vi "Double FFT Mesurament RT with Frequency Linearization & BackNoise Remove Test.vi"() -> ()   [LabVIEW 2014]
uses:
  <vilib>/Platform/TimedLoop/XDataNode/timing_clust.ctl
  <vilib>/Platform/TimedLoop/XDataNode/nitl_modes.ctl
  <vilib>/Platform/TimedLoop/XDataNode/wakeup.ctl
  <vilib>/FPGAPlugInAG/sbRIO-9636/niLvFpga_Open_sbRIO-9636.vi
  <vilib>/rvi/interface/common/dynamic/niFpgaDynamicAddResources.vi
  <vilib>/FPGAPlugInAG/Dynamic/niLvFpga_Reset_Dynamic.vi
  <vilib>/Utility/error.llb/Error Cluster From Error Code.vi
  <vilib>/rvi/errors/niLvFpgaAdjustHostInterfaceError.vi
  <vilib>/rvi/interface/common/niFpgaWaitOnOcc.vi
  <vilib>/FPGAPlugInAG/Dynamic/niLvFpga_Run_Dynamic.vi
  <vilib>/FPGAPlugInAG/Dynamic/niLvFpga_Abort_Dynamic.vi
  <vilib>/FPGAPlugInAG/Dynamic/niLvFpga_Close_Dynamic.vi
  <vilib>/rvi/interface/nirviOpenFPGA/nirviOpenFPGA.xnode
  FPGA Bitfiles/LaserDistanceSen_FPGATarget_DoubleFFTMesuram_6dDziXQAIGE.lvbitx
  FPGA Target/Test VIs/Double FFT Mesurament Test with Background Noise Remove.vi
  <vilib>/rvi/interface/nirviMethod/nirviMethod.xnode
  <vilib>/rvi/interface/nirviReadWriteControl/nirviReadWriteControl.xnode
  <vilib>/Platform/TimedLoop/XDataNode/XDataNode.xnode
  <vilib>/rvi/interface/nirviCloseFPGA/nirviCloseFPGA.xnode
  <vilib>/FPGAPlugInAG/Dynamic/niLvFpga_ConfigureFifo_Dynamic.vi
  <vilib>/rvi/errors/niLvFpgaMergeErrorWithErrorCode.vi
  <vilib>/FPGAPlugInAG/Dynamic/niLvFpga_StartFifo_Dynamic.vi
  <vilib>/rvi/interface/Simulation/niFpgaSimulationCallBeginRW.vi
  <vilib>/FPGAPlugInAG/Dynamic/niLvFpga_ReadFifo_Dynamic.vi
  <vilib>/Platform/TimedLoop/XDataNode/XDNodeRunTimeDep.lvlib
  NiFpgaLv.dll
panel:
  in  "polynomial order":i32=3
  in  "side points":i32=6
  out "2^(n-bit) misure mediate":dbl
  in  "n-bit":i32=10
  in  "SubtractionType":T1(ring)=enum."StartingCurve"
  out "Fondo Signal":dbl[](graph)
  in  "LowPass Filter: Low cutoff frequency":dbl=20000.0 format="%#_13g"
  in  "PolyFitting: Poly Grade":dbl=12.0
  in  "Scale Factor Rising":dbl=0.5
  out "2) Std Dev":dbl
  out "1) Std Dev":dbl
  in  "Scale Factor Falling":dbl=0.5
  in  "Triangolo dritto":bool
  in  "Acrive  Smooth":bool
  out "Complete SkewTri":dbl[](graph)
  out "2) Tri edge RISING":dbl[](graph)
  out "1) Tri edge FALLING":dbl[](graph)
  out "1) Ext Mean Time Curve":dbl[](graph)
  out "2) Ext Mean Time Curve":dbl[](graph)
  out "2) Mean Freq Curve Rising":dbl[](graph)
  out "1) Mean Freq Curve Falling":dbl[](graph)
  out "2) Freq curve":dbl[](graph)
  out "1) Freq curve":dbl[](graph)
  in  "FFT Sliding Win Size":i32=128
  out "1) SmoothSubSig":dbl[](graph)
  out "2) SmoothSubSig":dbl[](graph)
  in  "Acrive Fit":bool=TRUE
  in  "Poly Order":i32=3
  in  "Side points":i32=13
  in  "Poly Grade":dbl=5.0
  out "2) Signal&Fit 2":dbl[][](graph)
  out "1) Signal&Fit":dbl[][](graph)
  in  "tieni premuto per":i32=1
  out "Current Sig lin":i32
  in  "Acrive Linearization":bool
  in  "# Measurements for Linearization":i32=10
  in  "?":bool
  out "maxbin_secondFFT":i32
  out "maxbin_firstFFT":i32
  out "f_rise":dbl
  out "f_fall":dbl
  out "f_mean":dbl
  out "Velocity (m/s)":dbl
  out "Distance (m)":dbl
  in  "Initial Latency points":u32(slide)=400 scale=0.0..1249.0
  out "Second FFT (bin)":dbl[](graph)
  out "Second Signal (points) - Rising Triangular":dbl[](graph)
  out "First FFT (bin)":dbl[](graph)
  out "First Signal (points) - Falling Triangular":dbl[](graph)
  in  "Snapshot":bool
  in  "Windowing":T2(ring)=enum."Hanning"
  in  "first bin":i32=5
  in  "last bin":i32=255
  in  "lower limit 2":u32(slide)=738 scale=625.0..738.0
  in  "lower limit 1":u32(slide)=113 scale=0.0..113.0
  # "Estrazione del rumore di fondo (Background noise extraction)"
  # "Sav Golay Filter"
  # "WARNING:\nOnce pressed wait untill the end of operation"
  # "OFFLINE parameters"
  # "Triangolo storto\nda costante"
  # "Max Detection FFT bin range"
  # "ONLINE parameters"
  # "Se la sottrazione del fondo non è eseguita su FPGA.\n Attivarla per eseguirla lato RT"
  # "Smoothing (S-G Params)"
  # "Fitting"
  # "ONLY POWER OF 2"
  # "Min: 2 Max: 256 (2, 4, 8, 16, 32, 64, 128, 256)"
  # "LINEARIZATION FINAL RESULTS"
  # "dev standard (max-min)"
  # "%"
  # "%"
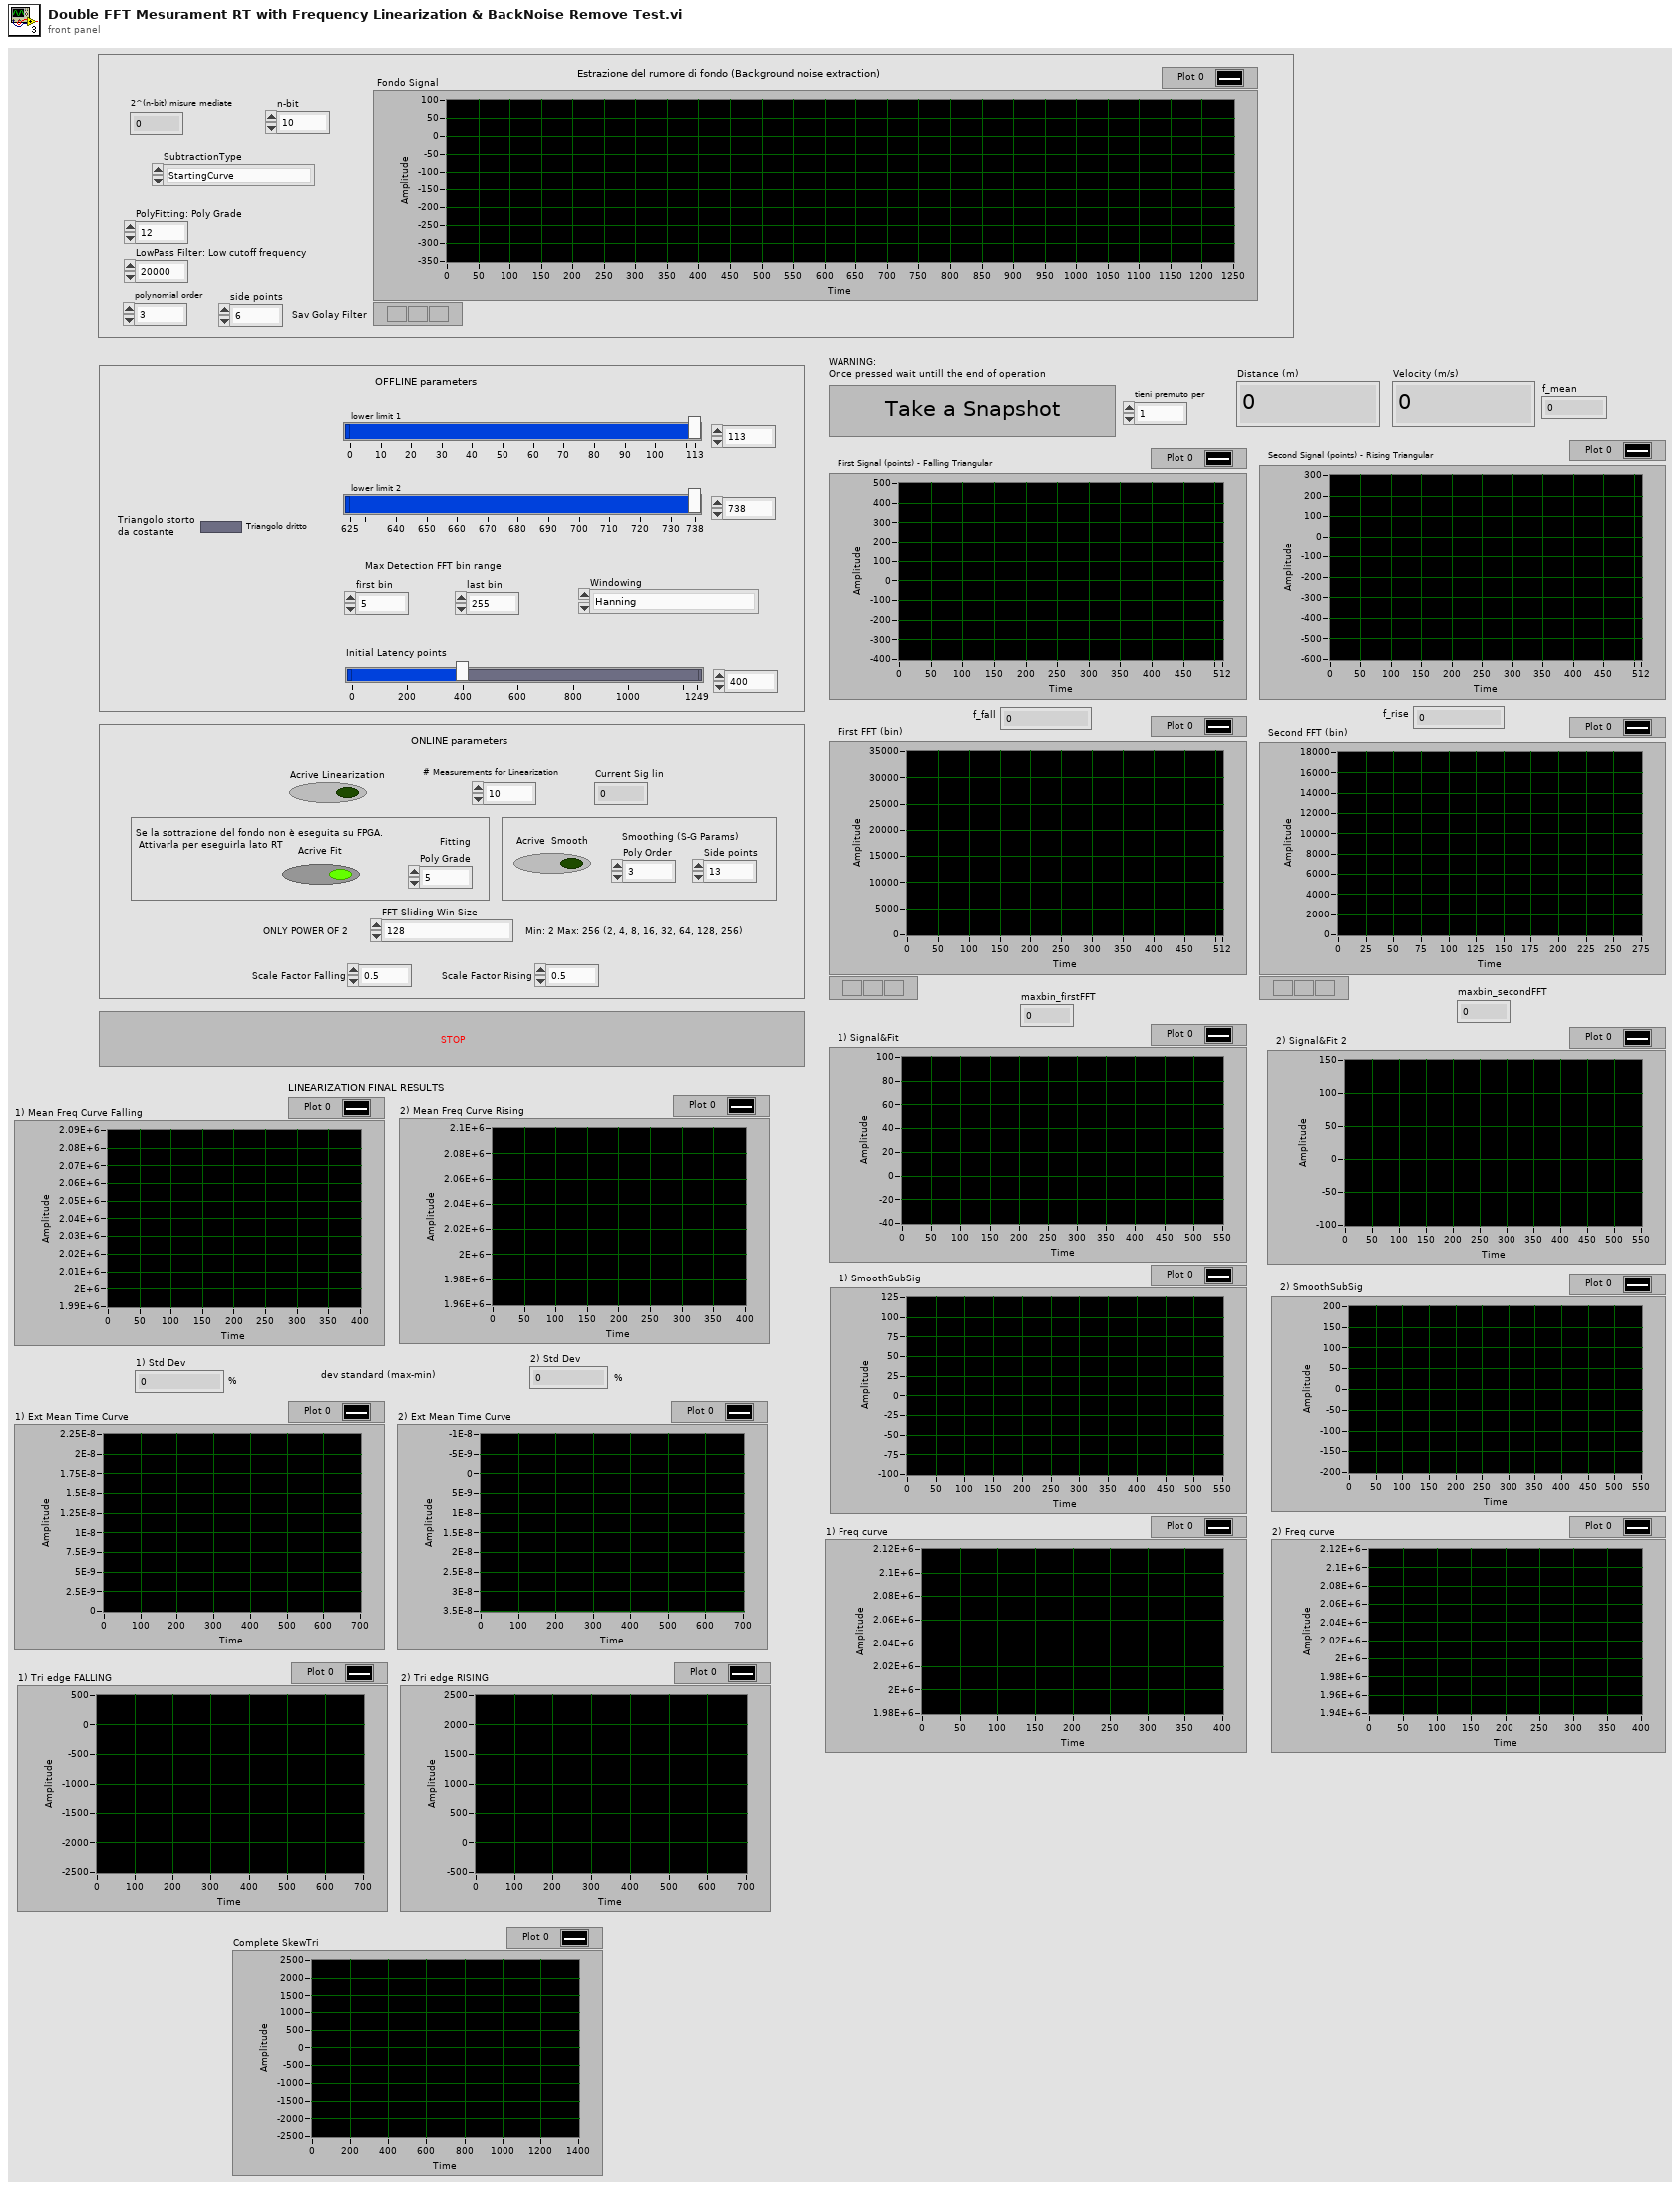
[diagram p1: front panel]
types:
  T1 = enum16{"NoSubtract", "StartingCurve", "LowPass", "PolyFitting", "SavGolay"}
  T2 = enum16{"None", "Hanning", "Hamming", "Blackman", "Blackman-Harris"}
  T3 = typedef "XDNodeRunTimeDep.lvlib/timing_clust.ctl" = cluster{"Expected End [f-1]":u64, "Actual End [f-1]":u64, "Finished Late? [f-1]":bool, "Expected End [i-1]":u64, "Actual End [i-1]":u64, "Finished Late? [i-1]":bool, "Expected Start [i]":u64, "Actual Start [i]":u64, "Expected Start [f]":u64, "Actual Start [f]":u64, "Source Name":string, "Structure Name":string, "Period":i64, "Deadline":i64, "Offset":i64, "Start":i64, "Priority":i32, "Timeout":i32, "Mode":T4, "Wakeup Reason":T5, "Error":errorcluster, "Source Type":string, "Secondary Source Type":string, "Global End Time":u64, "Global Start Time":u64, "Frame Duration":u64, "Iteration Duration":u64, "Assigned CPU":i32, "I/O Scan Engine Mode":u32}
  T4 = typedef "XDNodeRunTimeDep.lvlib/nitl_modes.ctl" = enum32{"No Change", "Process missed periods, maintain original phase", "Discard missed periods, maintain original phase", "Process missed periods, ignore original phase", "Discard missed periods, ignore original phase"}
  T5 = typedef "XDNodeRunTimeDep.lvlib/wakeup.ctl" = enum32{"Normal", "Aborted", "Asynchronous wakeup", "Timing source error", "Timed loop error", "Timeout"}
  T6 = typedef "NI_Matrix.lvlib/RealMatrix.ctl" = dbl[][]
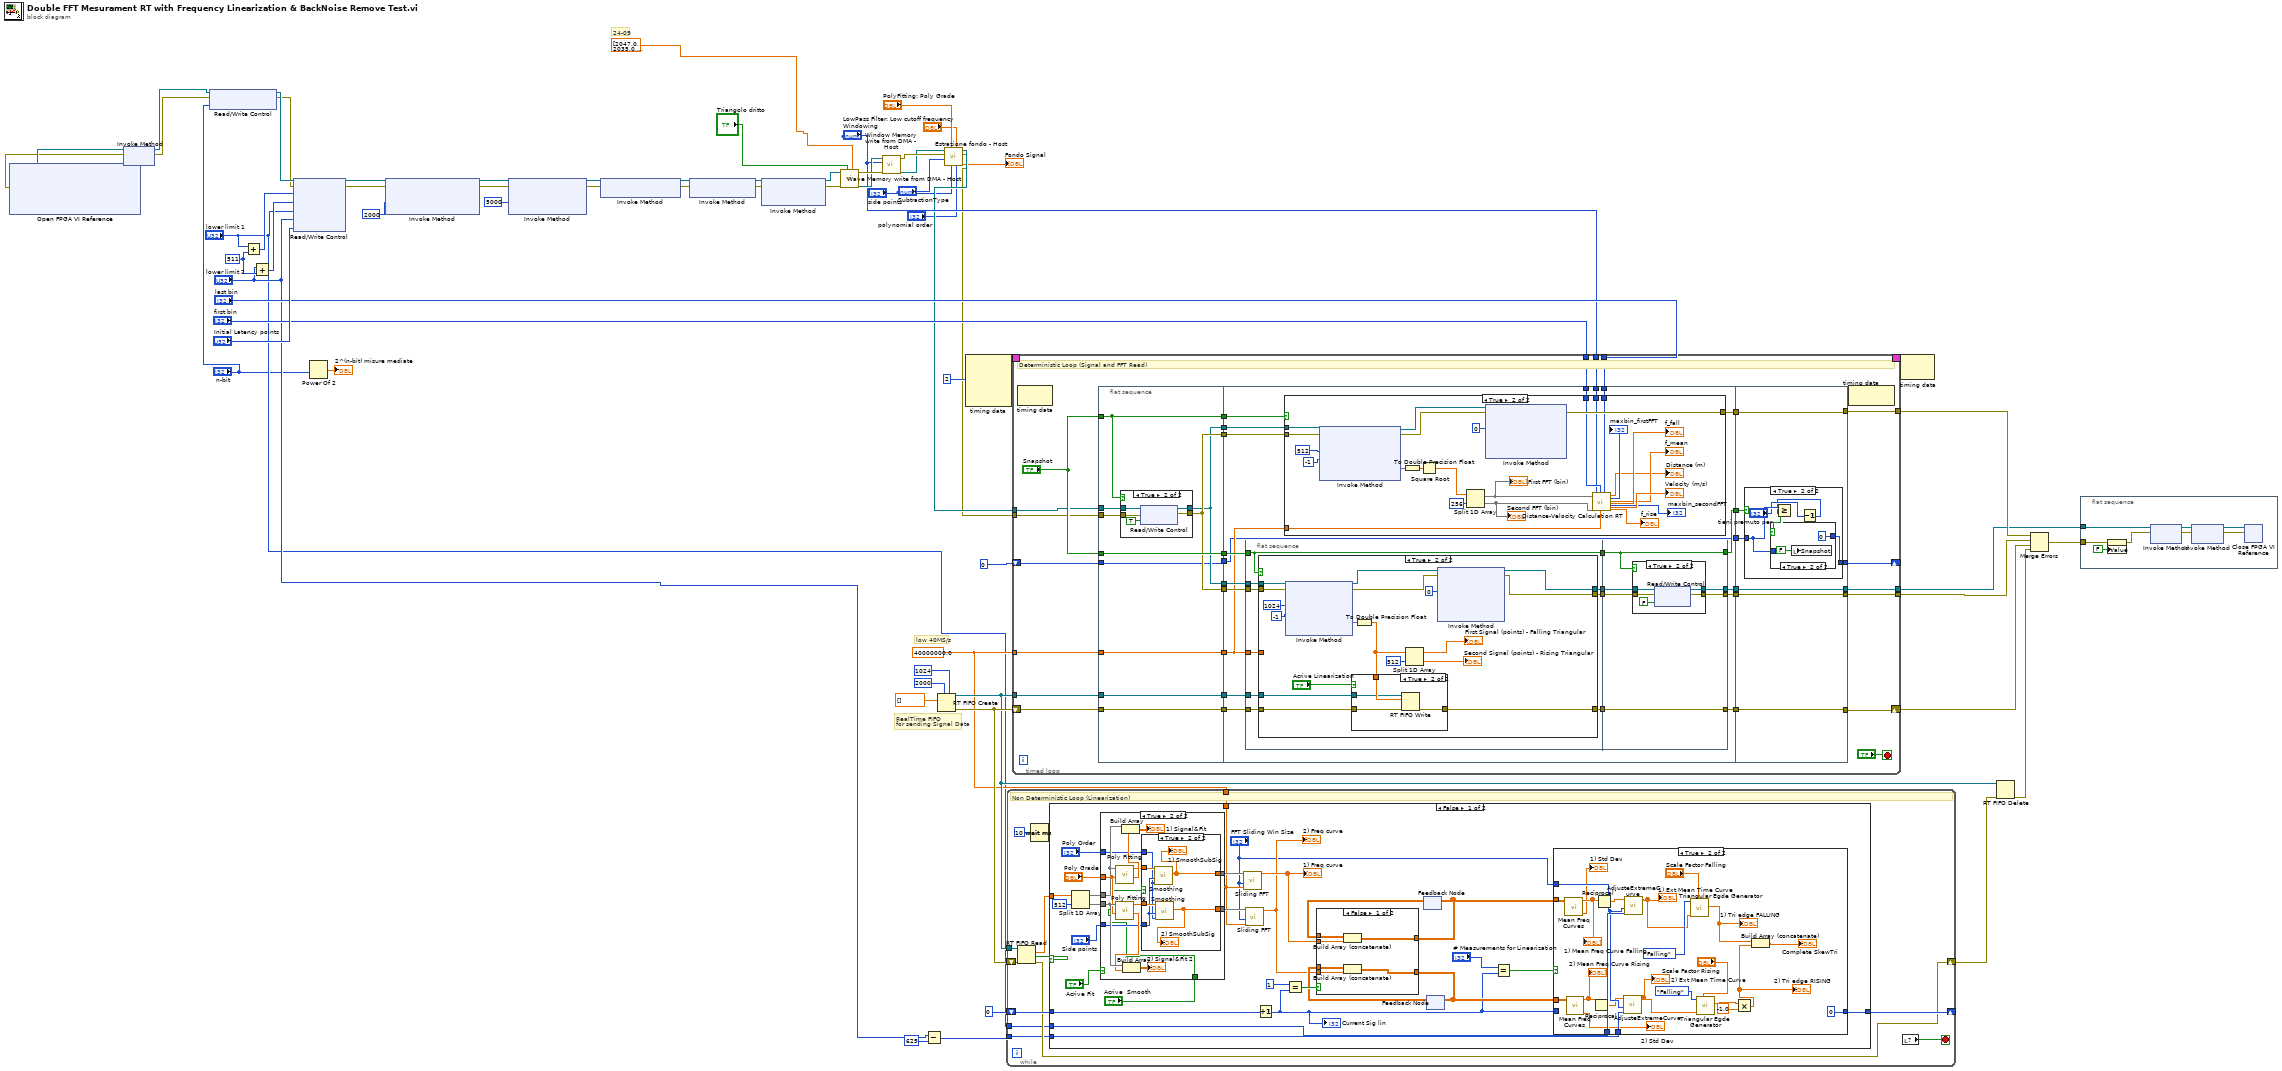
[diagram p0: block diagram]
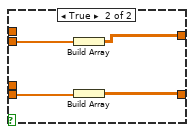
[diagram p5: hidden frame]
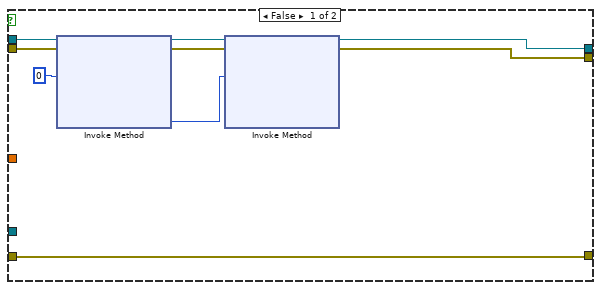
[diagram p8: hidden frame]
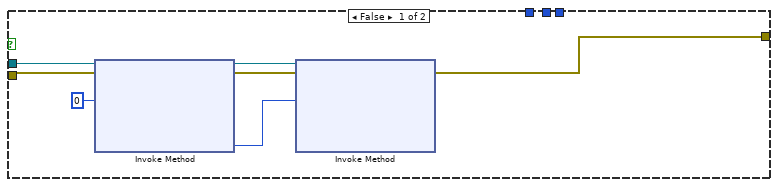
[diagram p11: hidden frame]
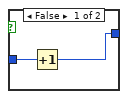
[diagram p13: hidden frame]
diagram:
  w63 = u32 511 ("y")
  w22 = 40000000.0 ("Sample Rate (S/s)")
  # "24-09"
  # "RealTime FIFO \nfor sending Signal Data"
  # "low 40MS/s"
  n1 = xnode "Open FPGA VI Reference"() -> ("FPGA VI Reference Out"=w8:refnum<k20>, "error out"=w7:errorcluster)  [unwired: 2 in]
  n2 = xnode "Invoke Method"("FPGA VI Reference In"=w8, "error in"=w7) -> ("FPGA VI Reference Out"=w5:refnum<k20>, "error out"=w3:errorcluster)
  n3 = xnode "Read/Write Control"("FPGA VI Reference In"=w5, "error in"=w3, "n-bit (2^nbit medie)"="n-bit") -> ("FPGA VI Reference Out"=w4:refnum<k20>, "error out"=w2:errorcluster)
  n4 = Add(x="lower limit 1", y=w63) -> (x+y=w65:u32)
  n5 = Add(x="lower limit 2", y=w63) -> (x+y=w64:u32)
  n6 = xnode "Read/Write Control"("FPGA VI Reference In"=w4, "error in"=w2, "upper limit 1"=w65, "upper limit 2"=w64, "lower limit 1"="lower limit 1", "lower limit 2"="lower limit 2", "Latency points"="Initial Latency points") -> ("FPGA VI Reference Out"=w62:refnum<k20>, "error out"=w61:errorcluster)
  n7 = Power Of 2(x="n-bit") -> (2^x=→"2^(n-bit) misure mediate":dbl)
  n8 = xnode "Invoke Method"("FPGA VI Reference In"=w62, "error in"=w61, "Requested Depth"=u32 2000) -> ("FPGA VI Reference Out"=w40:refnum<k20>, "error out"=w41:errorcluster)  [unwired: 1 out]
  n9 = xnode "Invoke Method"("FPGA VI Reference In"=w40, "error in"=w41, "Requested Depth"=u32 5000) -> ("FPGA VI Reference Out"=w54:refnum<k20>, "error out"=w55:errorcluster)  [unwired: 1 out]
  n10 = xnode "Invoke Method"("FPGA VI Reference In"=w54, "error in"=w55) -> ("FPGA VI Reference Out"=w38:refnum<k20>, "error out"=w39:errorcluster)
  n11 = xnode "Invoke Method"("FPGA VI Reference In"=w38, "error in"=w39) -> ("FPGA VI Reference Out"=w52:refnum<k20>, "error out"=w53:errorcluster)
  n12 = xnode "Invoke Method"("FPGA VI Reference In"=w52, "error in"=w53) -> ("FPGA VI Reference Out"=w58:refnum<k20>, "error out"=w57:errorcluster)  [unwired: 1 in]
  n13 = call "Wave Memory write from DMA - Host.vi"("Custom Triangular Signal (fal-ris)"=dbl[] [2047.0, 2035.0, 2022.0, 2010.0, 1997.0, 1985.0, 1972.0, 1960.0, 1948.0, 1935.0, 1923.0, 1911.0, 1899.0, 1886.0, 1874.0, 1862.0, 1850.0, 1838.0, 1825.0, 1813.0, 1801.0, 1789.0, 1777.0, 1765.0, 1753.0, 1741.0, 1729.0, 1717.0, 1705.0, 1693.0, 1681.0, 1669.0, 1657.0, 1645.0, 1634.0, 1622.0, 1610.0, 1598.0, 1586.0, 1575.0, 1563.0, 1551.0, 1540.0, 1528.0, 1516.0, 1505.0, 1493.0, 1481.0, 1470.0, 1458.0, 1447.0, 1435.0, 1424.0, 1412.0, 1401.0, 1389.0, 1378.0, 1366.0, 1355.0, 1344.0, 1332.0, 1321.0, 1310.0, 1298.0, 1287.0, 1276.0, 1265.0, 1253.0, 1242.0, 1231.0, 1220.0, 1209.0, 1198.0, 1186.0, 1175.0, 1164.0, 1153.0, 1142.0, 1131.0, 1120.0, 1109.0, 1098.0, 1087.0, 1076.0, 1065.0, 1055.0, 1044.0, 1033.0, 1022.0, 1011.0, 1000.0, 990.0, 979.0, 968.0, 958.0, 947.0, 936.0, 926.0, 915.0, 904.0, 894.0, 883.0, 873.0, 862.0, 852.0, 841.0, 831.0, 820.0, 810.0, 799.0, 789.0, 778.0, 768.0, 758.0, 747.0, 738.0, 727.0, 719.0, 712.0, 706.0, 700.0, 693.0, 687.0, 680.0, 674.0, 668.0, 661.0, 655.0, 648.0, 642.0, 636.0, 629.0, 623.0, 617.0, 610.0, 604.0, 598.0, 591.0, 584.0, 577.0, 569.0, 560.0, 552.0, 545.0, 538.0, 531.0, 525.0, 519.0, 512.0, 506.0, 500.0, 494.0, 488.0, 482.0, 476.0, 470.0, 464.0, 458.0, 452.0, 446.0, 436.0, 430.0, 424.0, 418.0, 412.0, 406.0, 400.0, 394.0, 388.0, 382.0, 376.0, 370.0, 364.0, 358.0, 352.0, 346.0, 338.0, 332.0, 325.0, 319.0, 313.0, 307.0, 301.0, 295.0, 290.0, 284.0, 278.0, 272.0, 267.0, 261.0, 255.0, 249.0, 244.0, 238.0, 232.0, 227.0, 221.0, 215.0, 209.0, 204.0, 198.0, 192.0, 187.0, 181.0, 175.0, 170.0, 164.0, 158.0, 153.0, 147.0, 141.0, 136.0, 130.0, 124.0, 119.0, 113.0, 108.0, 102.0, 96.0, 91.0, 85.0, 79.0, 74.0, 68.0, 62.0, 57.0, 51.0, 45.0, 39.0, 34.0, 28.0, 22.0, 16.0, 11.0, 5.0, 0.0, -6.0, -11.0, -17.0, -22.0, -28.0, -33.0, -39.0, -44.0, -50.0, -55.0, -61.0, -66.0, -72.0, -77.0, -83.0, -88.0, -94.0, -99.0, -105.0, -110.0, -116.0, -121.0, -127.0, -132.0, -137.0, -143.0, -148.0, -154.0, -159.0, -165.0, -170.0, -176.0, -181.0, -186.0, -192.0, -197.0, -203.0, -208.0, -214.0, -219.0, -224.0, -230.0, -235.0, -241.0, -246.0, -251.0, -257.0, -262.0, -268.0, -273.0, -278.0, -284.0, -289.0, -295.0, -300.0, -305.0, -311.0, -316.0, -321.0, -327.0, -332.0, -337.0, -343.0, -348.0, -354.0, -359.0, -364.0, -370.0, -375.0, -380.0, -386.0, -391.0, -397.0, -402.0, -407.0, -413.0, -418.0, -423.0, -429.0, -434.0, -439.0, -445.0, -450.0, -455.0, -461.0, -466.0, -471.0, -477.0, -482.0, -487.0, -493.0, -498.0, -503.0, -509.0, -514.0, -519.0, -525.0, -530.0, -535.0, -540.0, -546.0, -551.0, -556.0, -562.0, -567.0, -572.0, -578.0, -583.0, -588.0, -593.0, -599.0, -604.0, -609.0, -615.0, -620.0, -625.0, -630.0, -636.0, -641.0, -646.0, -651.0, -657.0, -662.0, -667.0, -673.0, -678.0, -683.0, -688.0, -694.0, -699.0, -704.0, -709.0, -715.0, -720.0, -725.0, -730.0, -736.0, -741.0, -746.0, -751.0, -757.0, -762.0, -767.0, -772.0, -778.0, -783.0, -788.0, -793.0, -799.0, -804.0, -809.0, -814.0, -820.0, -825.0, -830.0, -835.0, -841.0, -846.0, -851.0, -856.0, -862.0, -867.0, -872.0, -877.0, -883.0, -888.0, -893.0, -898.0, -903.0, -909.0, -914.0, -919.0, -924.0, -930.0, -935.0, -940.0, -945.0, -951.0, -956.0, -961.0, -966.0, -971.0, -977.0, -982.0, -987.0, -992.0, -998.0, -1003.0, -1008.0, -1013.0, -1018.0, -1024.0, -1029.0, -1034.0, -1039.0, -1045.0, -1050.0, -1055.0, -1060.0, -1065.0, -1071.0, -1076.0, -1081.0, -1086.0, -1092.0, -1097.0, -1102.0, -1107.0, -1112.0, -1118.0, -1123.0, -1128.0, -1133.0, -1138.0, -1144.0, -1149.0, -1154.0, -1159.0, -1165.0, -1170.0, -1175.0, -1180.0, -1185.0, -1191.0, -1196.0, -1201.0, -1206.0, -1211.0, -1217.0, -1222.0, -1227.0, -1232.0, -1237.0, -1243.0, -1248.0, -1253.0, -1258.0, -1263.0, -1269.0, -1274.0, -1279.0, -1284.0, -1289.0, -1295.0, -1300.0, -1305.0, -1310.0, -1315.0, -1321.0, -1326.0, -1331.0, -1336.0, -1341.0, -1347.0, -1352.0, -1357.0, -1362.0, -1367.0, -1373.0, -1378.0, -1383.0, -1388.0, -1393.0, -1399.0, -1404.0, -1409.0, -1414.0, -1419.0, -1425.0, -1430.0, -1435.0, -1440.0, -1445.0, -1450.0, -1456.0, -1461.0, -1466.0, -1471.0, -1476.0, -1482.0, -1487.0, -1492.0, -1497.0, -1502.0, -1508.0, -1513.0, -1518.0, -1523.0, -1528.0, -1534.0, -1539.0, -1544.0, -1549.0, -1554.0, -1560.0, -1565.0, -1570.0, -1575.0, -1580.0, -1586.0, -1591.0, -1596.0, -1601.0, -1606.0, -1612.0, -1617.0, -1622.0, -1627.0, -1632.0, -1637.0, -1643.0, -1648.0, -1653.0, -1658.0, -1663.0, -1669.0, -1674.0, -1679.0, -1684.0, -1689.0, -1695.0, -1700.0, -1705.0, -1710.0, -1715.0, -1721.0, -1726.0, -1731.0, -1736.0, -1741.0, -1747.0, -1752.0, -1757.0, -1762.0, -1767.0, -1773.0, -1778.0, -1783.0, -1788.0, -1793.0, -1799.0, -1804.0, -1809.0, -1814.0, -1819.0, -1825.0, -1830.0, -1835.0, -1840.0, -1845.0, -1851.0, -1856.0, -1861.0, -1866.0, -1871.0, -1876.0, -1882.0, -1887.0, -1892.0, -1897.0, -1902.0, -1908.0, -1913.0, -1918.0, -1923.0, -1928.0, -1934.0, -1939.0, -1944.0, -1949.0, -1954.0, -1960.0, -1965.0, -1970.0, -1975.0, -1980.0, -1986.0, -1991.0, -1996.0, -2001.0, -2006.0, -2012.0, -2017.0, -2022.0, -2027.0, -2032.0, -2038.0, -2043.0, -2048.0, -2047.0, -2037.0, -2027.0, -2017.0, -2007.0, -1997.0, -1987.0, -1977.0, -1967.0, -1957.0, -1947.0, -1937.0, -1927.0, -1917.0, -1907.0, -1897.0, -1888.0, -1878.0, -1868.0, -1858.0, -1848.0, -1838.0, -1828.0, -1819.0, -1809.0, -1799.0, -1789.0, -1780.0, -1770.0, -1760.0, -1750.0, -1741.0, -1731.0, -1721.0, -1712.0, -1702.0, -1692.0, -1683.0, -1673.0, -1663.0, -1654.0, -1644.0, -1635.0, -1625.0, -1615.0, -1606.0, -1596.0, -1587.0, -1577.0, -1568.0, -1558.0, -1549.0, -1539.0, -1530.0, -1520.0, -1511.0, -1501.0, -1492.0, -1483.0, -1473.0, -1464.0, -1454.0, -1445.0, -1436.0, -1426.0, -1417.0, -1408.0, -1398.0, -1389.0, -1380.0, -1371.0, -1361.0, -1352.0, -1343.0, -1334.0, -1324.0, -1315.0, -1306.0, -1297.0, -1288.0, -1278.0, -1269.0, -1260.0, -1251.0, -1242.0, -1233.0, -1224.0, -1215.0, -1205.0, -1196.0, -1187.0, -1178.0, -1169.0, -1160.0, -1151.0, -1142.0, -1133.0, -1124.0, -1115.0, -1106.0, -1097.0, -1088.0, -1080.0, -1071.0, -1062.0, -1053.0, -1044.0, -1035.0, -1026.0, -1017.0, -1009.0, -1000.0, -991.0, -982.0, -973.0, -965.0, -953.0, -944.0, -935.0, -920.0, -906.0, -889.0, -871.0, -854.0, -842.0, -834.0, -826.0, -818.0, -810.0, -802.0, -794.0, -786.0, -778.0, -770.0, -762.0, -754.0, -746.0, -739.0, -731.0, -723.0, -715.0, -707.0, -699.0, -690.0, -682.0, -672.0, -661.0, -651.0, -639.0, -627.0, -616.0, -606.0, -598.0, -591.0, -584.0, -577.0, -570.0, -563.0, -556.0, -549.0, -542.0, -535.0, -528.0, -520.0, -513.0, -506.0, -499.0, -492.0, -485.0, -478.0, -471.0, -464.0, -457.0, -451.0, -444.0, -437.0, -430.0, -423.0, -416.0, -409.0, -400.0, -390.0, -382.0, -373.0, -364.0, -356.0, -349.0, -343.0, -336.0, -330.0, -323.0, -317.0, -310.0, -304.0, -297.0, -291.0, -284.0, -278.0, -271.0, -265.0, -258.0, -252.0, -245.0, -239.0, -232.0, -226.0, -219.0, -213.0, -207.0, -200.0, -194.0, -187.0, -181.0, -175.0, -168.0, -162.0, -156.0, -149.0, -143.0, -136.0, -128.0, -121.0, -114.0, -107.0, -100.0, -93.0, -87.0, -80.0, -74.0, -68.0, -62.0, -56.0, -50.0, -44.0, -38.0, -32.0, -26.0, -20.0, -14.0, -8.0, -2.0, 5.0, 11.0, 17.0, 23.0, 29.0, 35.0, 41.0, 47.0, 53.0, 59.0, 65.0, 70.0, 76.0, 82.0, 88.0, 94.0, 100.0, 106.0, 112.0, 118.0, 124.0, 130.0, 136.0, 142.0, 148.0, 154.0, 161.0, 167.0, 174.0, 180.0, 186.0, 192.0, 198.0, 204.0, 210.0, 215.0, 221.0, 227.0, 233.0, 238.0, 244.0, 250.0, 255.0, 261.0, 267.0, 273.0, 278.0, 284.0, 290.0, 295.0, 301.0, 307.0, 312.0, 318.0, 324.0, 329.0, 335.0, 341.0, 346.0, 352.0, 358.0, 363.0, 369.0, 374.0, 380.0, 386.0, 391.0, 397.0, 402.0, 408.0, 414.0, 419.0, 425.0, 430.0, 436.0, 441.0, 447.0, 453.0, 458.0, 464.0, 470.0, 475.0, 481.0, 487.0, 493.0, 499.0, 504.0, 510.0, 516.0, 521.0, 527.0, 532.0, 538.0, 543.0, 549.0, 554.0, 560.0, 565.0, 571.0, 576.0, 582.0, 587.0, 593.0, 598.0, 604.0, 609.0, 614.0, 620.0, 625.0, 631.0, 636.0, 642.0, 647.0, 653.0, 658.0, 663.0, 669.0, 674.0, 680.0, 685.0, 691.0, 696.0, 701.0, 707.0, 712.0, 718.0, 723.0, 728.0, 734.0, 739.0, 745.0, 750.0, 755.0, 761.0, 766.0, 772.0, 777.0, 782.0, 788.0, 793.0, 798.0, 804.0, 809.0, 815.0, 820.0, 826.0, 831.0, 837.0, 842.0, 847.0, 853.0, 858.0, 863.0, 869.0, 874.0, 880.0, 885.0, 890.0, 895.0, 901.0, 906.0, 911.0, 917.0, 922.0, 927.0, 933.0, 938.0, 943.0, 948.0, 954.0, 959.0, 964.0, 970.0, 975.0, 980.0, 985.0, 991.0, 996.0, 1001.0, 1006.0, 1012.0, 1017.0, 1022.0, 1027.0, 1033.0, 1038.0, 1043.0, 1048.0, 1054.0, 1059.0, 1064.0, 1069.0, 1075.0, 1080.0, 1085.0, 1090.0, 1096.0, 1101.0, 1106.0, 1111.0, 1116.0, 1122.0, 1127.0, 1132.0, 1137.0, 1143.0, 1148.0, 1153.0, 1158.0, 1163.0, 1169.0, 1174.0, 1179.0, 1184.0, 1190.0, 1195.0, 1200.0, 1205.0, 1211.0, 1216.0, 1221.0, 1226.0, 1231.0, 1237.0, 1242.0, 1247.0, 1252.0, 1257.0, 1262.0, 1268.0, 1273.0, 1278.0, 1283.0, 1288.0, 1293.0, 1298.0, 1304.0, 1309.0, 1314.0, 1319.0, 1324.0, 1329.0, 1334.0, 1340.0, 1345.0, 1350.0, 1355.0, 1360.0, 1365.0, 1370.0, 1375.0, 1381.0, 1386.0, 1391.0, 1396.0, 1401.0, 1406.0, 1411.0, 1416.0, 1421.0, 1427.0, 1432.0, 1437.0, 1442.0, 1447.0, 1452.0, 1457.0, 1462.0, 1467.0, 1472.0, 1478.0, 1483.0, 1488.0, 1493.0, 1498.0, 1503.0, 1508.0, 1513.0, 1518.0, 1523.0, 1528.0, 1534.0, 1539.0, 1544.0, 1549.0, 1554.0, 1559.0, 1564.0, 1569.0, 1574.0, 1579.0, 1584.0, 1589.0, 1595.0, 1600.0, 1605.0, 1610.0, 1615.0, 1620.0, 1625.0, 1630.0, 1635.0, 1640.0, 1645.0, 1650.0, 1655.0, 1660.0, 1666.0, 1671.0, 1676.0, 1681.0, 1686.0, 1691.0, 1696.0, 1701.0, 1706.0, 1711.0, 1716.0, 1721.0, 1726.0, 1731.0, 1736.0, 1741.0, 1746.0, 1751.0, 1757.0, 1762.0, 1767.0, 1772.0, 1777.0, 1782.0, 1787.0, 1792.0, 1797.0, 1802.0, 1807.0, 1812.0, 1817.0, 1822.0, 1827.0, 1832.0, 1837.0, 1842.0, 1847.0, 1852.0, 1857.0, 1862.0, 1867.0, 1872.0, 1877.0, 1883.0, 1888.0, 1893.0, 1898.0, 1903.0, 1908.0, 1913.0, 1918.0, 1923.0, 1928.0, 1933.0, 1938.0, 1943.0, 1948.0, 1953.0, 1958.0, 1963.0, 1968.0, 1973.0, 1978.0, 1983.0, 1988.0, 1993.0, 1998.0, 2003.0, 2008.0, 2013.0, 2018.0, 2023.0, 2028.0, 2033.0, 2038.0, 2043.0, 2048.0] ("appended array"), "Triangolo dritto?"="Triangolo dritto", "error in"=w57, "FPGA VI Reference In"=w58) -> ("FPGA VI Reference Out"=w43:refnum<k20>, "error out"=w56:errorcluster)  [unwired: 5 in, 1 out]
  n14 = call "Window Memory write from DMA - Host.vi"("error in"=w56, "Enum"="Windowing", "FPGA VI Reference In"=w43) -> ("FPGA VI Reference Out"=w18:refnum<k20>, "error out"=w19:errorcluster)  [unwired: 5 in, 2 out]
  n15 = Subtract(x="lower limit 2", y=u32 625) -> (x-y=w24:u32)
  n16 = RT FIFO Create(1:dbl[] [] ("double precision float"), 4:u32 2000 ("size (10)"), 6:u32 1024 ("elements in array (1)")) -> (8:w30:refnum<k33>, 11:w32:errorcluster)  [unwired: 5 in, 1 out]
  n17 = call "Estrazione fondo - Host.vi"("polynomial order"="polynomial order", "LowPass Filter: Low cutoff frequency"="LowPass Filter: Low cutoff frequency", "side points"="side points", "PolyFitting: Poly Grade"="PolyFitting: Poly Grade", "SubtractionType"="SubtractionType", "error in"=w19, "FPGA VI Reference In"=w18) -> ("Fondo Signal"=→"Fondo Signal":dbl[], "error out"=w16:errorcluster, "FPGA VI Reference Out"=w17:refnum<k20>)  [unwired: 1 in, 1 out]
  n18 = node-c288(i64 2 ("Period")) -> (w51:T3)  [unwired: 3 in]
  n19 = while {
    shift-right: [w69] -> w29
    shift-left: w32 -> [w71]
    tunnel: w30 -> [w76]
    shift-right: [w70] -> _
    shift-left: 0 -> [w74]
    tunnel: "lower limit 1" -> [w66]
    tunnel: w24 -> [w67]
    tunnel: w22 -> [w68]
    stop <- w75 stop-if-true
    # "Non Deterministic Loop (Linearization)"
    n20 = RT FIFO Read(0:w76, 3:w71) -> (9:w73:dbl[], 10:w72:bool, 11:w69:errorcluster)  [unwired: 2 in, 2 out]
    n21 = Wait (ms)(milliseconds to wait=u32 10 ("millisecond multiple")) -> ()  [unwired: 1 out]
    n22 = case shown="False" w72 {
      tunnel: w74 -> [w105 w164]
      tunnel: [w94 w164] -> w70
      tunnel: w73 -> [w103 _]
      tunnel: w68 -> [w84 _]
      tunnel: w67 -> [w81 _]
      tunnel: w66 -> [w80 _]
      frame False {
        n23 = Split 1D Array(array=w103, index=512) -> (first subarray=w92:dbl[], second subarray=w91:dbl[])
        n24 = case shown="True" "Acrive Fit" {
          tunnel: w92 -> [w107 w121]
          tunnel: w91 -> [w106 w117]
          tunnel: "Poly Grade" -> [_ w113]
          tunnel: "Side points" -> [_ w112]
          tunnel: "Poly Order" -> [_ w111]
          tunnel: [w106 w110] -> w85
          tunnel: [w107 w108] -> w86
          tunnel: "Acrive  Smooth" -> [_ w109]
          frame False {
          }
          frame True {
            n25 = call "Poly Fitting.vi"("Poly Grade"=w113, "Signal"=w121) -> ("Poly Signal"=w120:dbl[], "SubtractedSignal"=w115:dbl[])  [unwired: 8 in]
            n26 = call "Poly Fitting.vi"("Poly Grade"=w113, "Signal"=w117) -> ("Poly Signal"=w116:dbl[], "SubtractedSignal"=w114:dbl[])  [unwired: 8 in]
            n27 = Build Array(w121, w120) -> (→"1) Signal&Fit":dbl[][])
            n28 = Build Array(w117, w116) -> (→"2) Signal&Fit 2":dbl[][])
            n29 = case shown="True" w109 {
              tunnel: w115 -> [w123 w129]
              tunnel: w114 -> [w122 w128]
              tunnel: w112 -> [_ w127]
              tunnel: w111 -> [_ w126]
              tunnel: [w122 w125] -> w110
              tunnel: [w123 w124] -> w108
              frame False {
              }
              frame True {
                n30 = call "Smoothing.vi"("polynomial order"=w126, "side points"=w127, "SubtractedSignal"=w129) -> ("SubSmoothSignal"=w124:dbl[])  [unwired: 8 in]
                "1) SmoothSubSig" <- w124
                n31 = call "Smoothing.vi"("polynomial order"=w126, "side points"=w127, "SubtractedSignal"=w128) -> ("SubSmoothSignal"=w125:dbl[])  [unwired: 8 in]
                "2) SmoothSubSig" <- w125
              }
            }
          }
        }
        n32 = call "Sliding FFT.vi"("Sample Freq"=w84, "FFT Win Size"="FFT Sliding Win Size", "SubSmoothSignal"=w86) -> ("Freq samples"=w83:dbl[])  [unwired: 7 in, 1 out]
        "1) Freq curve" <- w83
        n33 = call "Sliding FFT.vi"("Sample Freq"=w84, "FFT Win Size"="FFT Sliding Win Size", "SubSmoothSignal"=w85) -> ("Freq samples"=w82:dbl[])  [unwired: 7 in, 1 out]
        "2) Freq curve" <- w82
        n34 = Increment(x=w105) -> (x+1=w95:i32)
        "Current Sig lin" <- w95
        n35 = Equal?(x=1, y=w95) -> (x = y?=w101:bool)
        n36 = feedback #1() -> (w100:T6)  [unwired: 1 in]
        n37 = feedback #2() -> (w99:T6)  [unwired: 1 in]
        n38 = case shown="False" w101 {
          tunnel: w82 -> [w158 w161]
          tunnel: w83 -> [w159 w163]
          tunnel: [w157 w160] -> w96
          tunnel: [w156 w162] -> w97
          tunnel: w100 -> [w155 _]
          tunnel: w99 -> [w154 _]
          frame False {
            n39 = Build Array (concatenate)(w155, w159) -> (w156:T6)
            n40 = Build Array (concatenate)(w154, w158) -> (w157:T6)
          }
          frame True {
            n41 = Build Array(w163) -> (w162:T6)
            n42 = Build Array(w161) -> (w160:T6)
          }
        }
        n43 = feedback-in #1(w97) -> ()
        n44 = feedback-in #2(w96) -> ()
        n45 = Equal?(x="# Measurements for Linearization", y=w95) -> (x = y?=w93:bool)
        n46 = case shown="True" w93 {
          tunnel: w97 -> [_ w132]
          tunnel: w96 -> [_ w131]
          tunnel: w95 -> [w130 _]
          tunnel: [w130 0] -> w94
          tunnel: w81 -> [_ w148]
          tunnel: w80 -> [_ w147]
          tunnel: "FFT Sliding Win Size" -> [_ w146]
          frame False {
          }
          frame True {
            n47 = call "Mean Freq Curves.vi"("Set of Freq samples"=w132) -> ("StdDev%"=→"1) Std Dev":dbl, "Mean Freq Curve"=w141:dbl[])  [unwired: 9 in]
            "1) Mean Freq Curve Falling" <- w141
            n48 = call "Mean Freq Curves.vi"("Set of Freq samples"=w131) -> ("StdDev%"=→"2) Std Dev":dbl, "Mean Freq Curve"=w143:dbl[])  [unwired: 9 in]
            "2) Mean Freq Curve Rising" <- w143
            n49 = Reciprocal(x=w143) -> (1/x=w142:dbl[])
            n50 = Reciprocal(x=w141) -> (1/x=w140:dbl[])
            n51 = call "AdjusteExtremeCurve.vi"("Init Bins Discarded"=w148, "FFT Size Window"=w146, "Freq sample"=w142) -> ("Extended Freq Sample"=w144:dbl[])  [unwired: 8 in]
            "2) Ext Mean Time Curve" <- w144
            n52 = call "AdjusteExtremeCurve.vi"("Init Bins Discarded"=w147, "FFT Size Window"=w146, "Freq sample"=w140) -> ("Extended Freq Sample"=w145:dbl[])  [unwired: 8 in]
            "1) Ext Mean Time Curve" <- w145
            n53 = call "Triangular Egde Generator.vi"("fattore"="Scale Factor Falling", "Sample values"=w145, "Triangular edge"=enum16{"Rising", "Falling"}."Falling") -> ("Skew Triangular"=w150:dbl[])  [unwired: 8 in]
            "1) Tri edge FALLING" <- w150
            n54 = call "Triangular Egde Generator.vi"("fattore"="Scale Factor Rising", "Sample values"=w144, "Triangular edge"=enum16{"Rising", "Falling"}."Falling") -> ("Skew Triangular"=w138:dbl[])  [unwired: 8 in]
            n55 = Multiply(x=w138, y=-1.0) -> (x*y=w137:dbl[])
            "2) Tri edge RISING" <- w137
            n56 = Build Array (concatenate)(w150, w137) -> (→"Complete SkewTri":dbl[])
          }
        }
      }
      frame True {
      }
    }
    n57 = local read item#18() -> (w75:bool)
  }
  n58 = timed-loop {
    tunnel: w17 -> [w191]
    tunnel: w16 -> [w192]
    tunnel: [w194] -> w48
    tunnel: w22 -> [w196]
    tunnel: [w195] -> w47
    timing: w51 -> [_]
    timing-out: [_] -> w50
    tunnel: "first bin" -> [w180]
    tunnel: "last bin" -> [w179]
    tunnel: [w177] -> w42
    tunnel: "Windowing" -> [w175]
    shift-right: [w169] -> w33
    shift-left: w32 -> [w171]
    tunnel: w30 -> [w173]
    shift-right: [w165] -> _
    shift-left: 0 -> [w167]
    stop <- "?" stop-if-true
    # "Deterministic Loop (Signal and FFT Read)"
    n59 = node-c288() -> ()  [unwired: 1 in, 1 out]
    n60 = flat-sequence {
      tunnel: w191 -> [w204]
      tunnel: w192 -> [w205]
      tunnel: "Snapshot" -> [w202]
      tunnel: "Snapshot" -> [w207]
      tunnel: w196 -> [w208]
      tunnel: [w206] -> w190
      tunnel: [w208] -> w189
      tunnel: [w207] -> w188
      tunnel: [w202] -> w187
      tunnel: [w206] -> w186
      tunnel: [w203] -> w185
      tunnel: [w203] -> w184
      tunnel: [w201] -> w174
      tunnel: w173 -> [w201]
      tunnel: [w200] -> w172
      tunnel: w171 -> [w200]
      tunnel: [w199] -> w168
      tunnel: w167 -> [w199]
      tunnel: w190 -> [w233]
      tunnel: w189 -> [w221]
      tunnel: w188 -> [w227]
      tunnel: w187 -> [w230]
      tunnel: w186 -> [w229]
      tunnel: w185 -> [w228]
      tunnel: w184 -> [w234]
      tunnel: [w232] -> w183
      tunnel: [w231] -> w182
      tunnel: [w226] -> w181
      tunnel: w180 -> [w225]
      tunnel: w179 -> [w224]
      tunnel: [w223] -> w176
      tunnel: w175 -> [w222]
      tunnel: w174 -> [w220]
      tunnel: w172 -> [w219]
      tunnel: [w217] -> w170
      tunnel: w168 -> [w216]
      tunnel: [w216] -> w166
      tunnel: [w329] -> w194
      tunnel: [w330] -> w195
      tunnel: w183 -> [w330]
      tunnel: w182 -> [w329]
      tunnel: w181 -> [w328]
      tunnel: [w327] -> w177
      tunnel: w176 -> [w327]
      tunnel: [w326] -> w169
      tunnel: w170 -> [w326]
      tunnel: w166 -> [w325]
      tunnel: [w324] -> w165
      frame #0 {
        n61 = case shown="True" w202 {
          tunnel: [w209 w214] -> w206
          tunnel: w205 -> [w209 w213]
          tunnel: w204 -> [w210 w212]
          tunnel: [w210 w211] -> w203
          frame False {
          }
          frame True {
            n62 = xnode "Read/Write Control"("FPGA VI Reference In"=w212, "error in"=w213, "snapshot"=TRUE) -> ("FPGA VI Reference Out"=w211:refnum<k20>, "error out"=w214:errorcluster)
          }
        }
      }
      frame #1 {
        n63 = flat-sequence {
          tunnel: w234 -> [w246]
          tunnel: w233 -> [w245]
          tunnel: w221 -> [w244]
          tunnel: w227 -> [w241]
          tunnel: [w243] -> w237
          tunnel: [w242] -> w236
          tunnel: [w241] -> w235
          tunnel: w220 -> [w240]
          tunnel: w219 -> [w239]
          tunnel: [w238] -> w218
          tunnel: [w282] -> w231
          tunnel: w237 -> [w284]
          tunnel: w236 -> [w283]
          tunnel: w235 -> [w281]
          tunnel: [w281] -> w226
          tunnel: [w280] -> w223
          tunnel: [w279] -> w217
          tunnel: w218 -> [w279]
          frame #0 {
            n64 = case shown="True" w241 {
              tunnel: w246 -> [w254 w273]
              tunnel: w245 -> [w252 w272]
              tunnel: [w251 w265] -> w242
              tunnel: w244 -> [_ _]
              tunnel: [w248 w264] -> w243
              tunnel: w240 -> [_ w259]
              tunnel: w239 -> [w247 w258]
              tunnel: [w247 w257] -> w238
              frame False {
                n65 = xnode "Invoke Method"("FPGA VI Reference In"=w254, "error in"=w252, "Number of Elements"=u32 0) -> ("FPGA VI Reference Out"=w250:refnum<k20>, "error out"=w249:errorcluster, "Elements Remaining"=w253:u32)  [unwired: 1 in, 1 out]
                n66 = xnode "Invoke Method"("FPGA VI Reference In"=w250, "error in"=w249, "Number of Elements"=w253) -> ("FPGA VI Reference Out"=w248:refnum<k20>, "error out"=w251:errorcluster)  [unwired: 1 in, 2 out]
              }
              frame True {
                n67 = xnode "Invoke Method"("FPGA VI Reference In"=w273, "error in"=w272, "Number of Elements"=u32 1024, "Timeout (ms)"=-1) -> ("FPGA VI Reference Out"=w267:refnum<k20>, "error out"=w266:errorcluster, "Data"=w269:fxp<+/-,12,12>[])  [unwired: 1 out]
                n68 = To Double Precision Float(number=w269) -> (double precision float=w260:dbl[])
                n69 = case shown="True" "Acrive Linearization" {
                  tunnel: w260 -> [_ w278]
                  tunnel: w259 -> [_ w277]
                  tunnel: w258 -> [w274 w276]
                  tunnel: [w274 w275] -> w257
                  frame False {
                  }
                  frame True {
                    n70 = RT FIFO Write(0:w277, 1:w278, 3:w276) -> (11:w275:errorcluster)  [unwired: 2 in, 3 out]
                  }
                }
                n71 = Split 1D Array(array=w260, index=512) -> (first subarray=→"First Signal (points) - Falling Triangular":dbl[], second subarray=→"Second Signal (points) - Rising Triangular":dbl[])
                n72 = xnode "Invoke Method"("FPGA VI Reference In"=w267, "error in"=w266, "Number of Elements"=u32 0) -> ("FPGA VI Reference Out"=w264:refnum<k20>, "error out"=w265:errorcluster)  [unwired: 1 in, 2 out]
              }
            }
          }
          frame #1 {
            n73 = case shown="True" w281 {
              tunnel: [w286 w289] -> w282
              tunnel: w284 -> [w285 w290]
              tunnel: w283 -> [w286 w288]
              tunnel: [w285 w287] -> w280
              frame False {
              }
              frame True {
                n74 = xnode "Read/Write Control"("FPGA VI Reference In"=w290, "error in"=w288, "snapshot"=FALSE) -> ("FPGA VI Reference Out"=w287:refnum<k20>, "error out"=w289:errorcluster)
              }
            }
          }
        }
        n75 = case shown="True" w230 {
          tunnel: w228 -> [w297 w318]
          tunnel: w229 -> [w294 w319]
          tunnel: [w293 w317] -> w232
          tunnel: w225 -> [_ w304]
          tunnel: w224 -> [_ w305]
          tunnel: w222 -> [_ w301]
          tunnel: w221 -> [_ w299]
          frame False {
            n76 = xnode "Invoke Method"("FPGA VI Reference In"=w297, "error in"=w294, "Number of Elements"=u32 0) -> ("FPGA VI Reference Out"=w295:refnum<k20>, "error out"=w292:errorcluster, "Elements Remaining"=w296:u32)  [unwired: 1 in, 1 out]
            n77 = xnode "Invoke Method"("FPGA VI Reference In"=w295, "error in"=w292, "Number of Elements"=w296) -> ("error out"=w293:errorcluster)  [unwired: 1 in, 3 out]
          }
          frame True {
            n78 = xnode "Invoke Method"("FPGA VI Reference In"=w318, "error in"=w319, "Number of Elements"=u32 512, "Timeout (ms)"=-1) -> ("FPGA VI Reference Out"=w315:refnum<k20>, "error out"=w316:errorcluster, "Data"=w321:fxp<+,44,44>[])  [unwired: 1 out]
            n79 = To Double Precision Float(number=w321) -> (double precision float=w320:dbl[])
            n80 = Square Root(x=w320) -> (sqrt(x)=w313:dbl[])
            n81 = Split 1D Array(array=w313, index=256) -> (first subarray=w311:dbl[], second subarray=w310:dbl[])
            "First FFT (bin)" <- w311
            "Second FFT (bin)" <- w310
            n82 = xnode "Invoke Method"("FPGA VI Reference In"=w315, "error in"=w316, "Number of Elements"=u32 0) -> ("error out"=w317:errorcluster)  [unwired: 1 in, 3 out]
            n83 = call "Distance-Velocity Calculation RT.vi"("First FFT"=w311, "Second FFT"=w310, "Windowing"=w301, "first FFT bin"=w304, "Sample Rate (S/s)"=w299, "last FFT bin"=w305) -> ("F_rise"=→"f_rise":dbl, "maxbin_firstFFT"=→"maxbin_firstFFT":i32, "maxbin_secondFFT"=→"maxbin_secondFFT":i32, "Distance (m)"=→"Distance (m)":dbl, "f_mean"=→"f_mean":dbl, "F_fall"=→"f_fall":dbl, "Velocity (m/s)"=→"Velocity (m/s)":dbl)  [unwired: 7 in]
          }
        }
      }
      frame #2 {
        n84 = case shown="True" w328 {
          tunnel: w325 -> [w331 w335]
          tunnel: [w331 w336] -> w324
          frame False {
          }
          frame True {
            n85 = Decrement(x="tieni premuto per") -> (x-1=w332:i32)
            n86 = Greater Or Equal?(x=w335, y=w332) -> (x >= y?=w334:bool)
            n87 = case shown="True" w334 {
              tunnel: w335 -> [w337 _]
              tunnel: [w338 0] -> w336
              frame False {
                n88 = Increment(x=w337) -> (x+1=w338:i32)
              }
              frame True {
                n89 = local write "Snapshot"(FALSE ("Snapshot")) -> ()
              }
            }
          }
        }
      }
    }
    n90 = node-c288() -> ()  [unwired: 1 in, 1 out]
  }
  n91 = node-c288(w50) -> ()  [unwired: 1 out]
  n92 = RT FIFO Delete(0:w30, 3:w29) -> (11:w28:errorcluster)  [unwired: 1 in]
  n93 = Merge Errors(w47, w48, w33, w28) -> (w31:errorcluster)
  n94 = flat-sequence {
    tunnel: w31 -> [w344]
    tunnel: w42 -> [w341]
    frame #0 {
      n95 = property class="Bool (strict)"(error in=w344, "Value"=FALSE ("stop")) -> (error out=w343:errorcluster)  [unwired: 1 in, 1 out]
      n96 = xnode "Invoke Method"("FPGA VI Reference In"=w341, "error in"=w343) -> ("FPGA VI Reference Out"=w346:refnum<k20>, "error out"=w345:errorcluster)
      n97 = xnode "Invoke Method"("FPGA VI Reference In"=w346, "error in"=w345) -> ("FPGA VI Reference Out"=w347:refnum<k20>, "error out"=w348:errorcluster)
      n98 = xnode "Close FPGA VI Reference"("FPGA VI Reference In"=w347, "error in"=w348) -> ()  [unwired: 1 out]
    }
  }
